vi "Add Address Map Element.vi"(0 "niInstr AXI4-Lite address space collection v1 FPGA in":refnum<class "niInstr AXI4-Lite Address Space Collection v1 FPGA.lvclass">, 5 "address map element in":T1) -> (4 "niInstr AXI4-Lite address space collection v1 FPGA out":refnum<class "niInstr AXI4-Lite Address Space Collection v1 FPGA.lvclass">)   [LabVIEW 2015, in "niInstr AXI4-Lite Address Space Collection v1 FPGA.lvclass"]
doc: "Adds the specified Address Map Element to the Address Space Collection.\n\n<B>Input Parameters</B>\n\n<B>niInstr AXI4-Lite address space collection v1 FPGA in</B> is a reference to the Address Space Collection passed in from the previous VI.\n\n<B>address map element in</B> contains information related to a specific address map.\n\n<B>address map element in.UID</B> is the unique identifier of the address map element.\n\n<B>address map element in.version</B> is the version of the address map element.\n\n<B>address map element in.oldest compatible version</B> is the oldest version of the address map that is compatible with the current version.\n\n<B>address map element in.instance</B> is the specific instance of the specified address map.\n\n<B>address map element in.number of children</B> is the number of address map elements which are children of the current address map element.\n\n<B>address map element in.offset</B> is the register offset of the Address Map Element on the hardware.\n\n<B>Output Parameters</B>\n\n<B>niInstr AXI4-Lite address space collection v1 FPGA out</B> passes a reference to the Address Space Collection to the next VI."
uses:
  <instrlib>/_niInstr/CLIP Adapters/v1/FPGA/AXI4-Lite/Address Space Collection/niInstr AXI4-Lite Address Space Collection v1 FPGA.lvclass
  <instrlib>/_niInstr/Instruction Framework/v1/FPGA/Typedefs/Address Map Element.ctl
  <instrlib>/_niInstr/CLIP Adapters/v1/FPGA/AXI4-Lite/Address Space Collection/niInstr AXI4-Lite Address Space Collection v1 FPGA.lvclass/niInstr AXI4-Lite Address Space Collection v1 FPGA.ctl
  <instrlib>/_niInstr/CLIP Adapters/v1/FPGA/AXI4-Lite/Address Space/niInstr AXI4-Lite Address Space v1 FPGA.lvclass
  <instrlib>/_niInstr/Instruction Framework/v1/FPGA/Typedefs/niInstr Instruction Framework v1 FPGA.lvlib
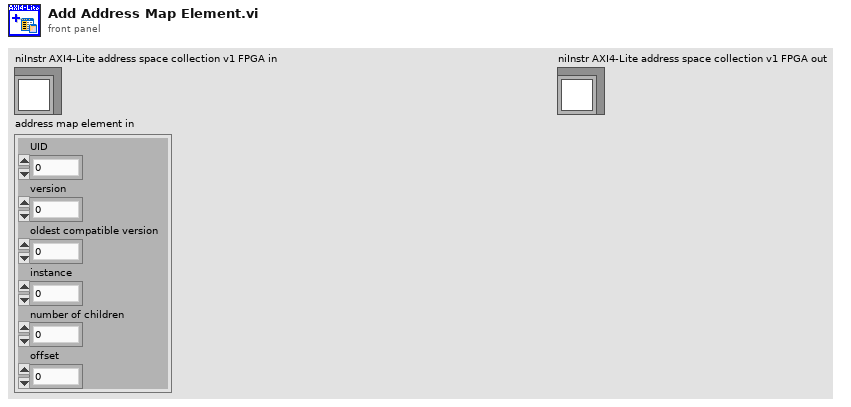
[diagram p1: front panel]
types:
  T1 = typedef "niInstr Instruction Framework v1 FPGA.lvlib/Address Map Element.ctl" = cluster{"UID":u16, "version":u16, "oldest compatible version":u16, "instance":u8, "number of children":u8, "offset":u32}
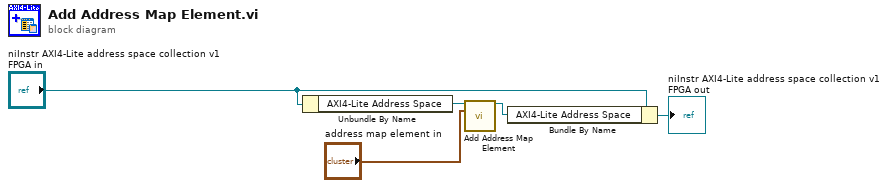
[diagram p0: block diagram]
diagram:
  n1 = Unbundle By Name("niInstr AXI4-Lite address space collection v1 FPGA in") -> ("AXI4-Lite Address Space"=w3:refnum<class "niInstr AXI4-Lite Address Space v1 FPGA.lvclass">)
  n2 = call <instrlib>:"Add Address Map Element.vi"("niInstr AXI4-Lite address space v1 FPGA in"=w3, "address map element in"="address map element in") -> ("niInstr AXI4-Lite address space v1 FPGA out"=w2:refnum<class "niInstr AXI4-Lite Address Space v1 FPGA.lvclass">)  [unwired: 13 in]
  n3 = Bundle By Name(cluster="niInstr AXI4-Lite address space collection v1 FPGA in", "AXI4-Lite Address Space"=w2) -> (→"niInstr AXI4-Lite address space collection v1 FPGA out":refnum<class "niInstr AXI4-Lite Address Space Collection v1 FPGA.lvclass">)
